vi "arrays.vi"() -> ()   [LabVIEW 2023]
panel:
  out "Waveform Chart":cluster{dbl, dbl}(graph)
  in  "stop":bool
  out "Waveform Graph":dbl[](graph)
  out "Array 4":dbl[][](array[numeric])
  out "Array 3":dbl[](array[numeric])
  in  "Array 2":dbl[](array[numeric])
  out "Array":dbl[](array[numeric])
  out "x+y 4":dbl[](array[numeric])
  out "x+y 3":dbl[](array[numeric])
  out "x+y 2":dbl[](array[numeric])
  out "x+y":dbl
  out "initialized array":dbl[][](array[numeric])
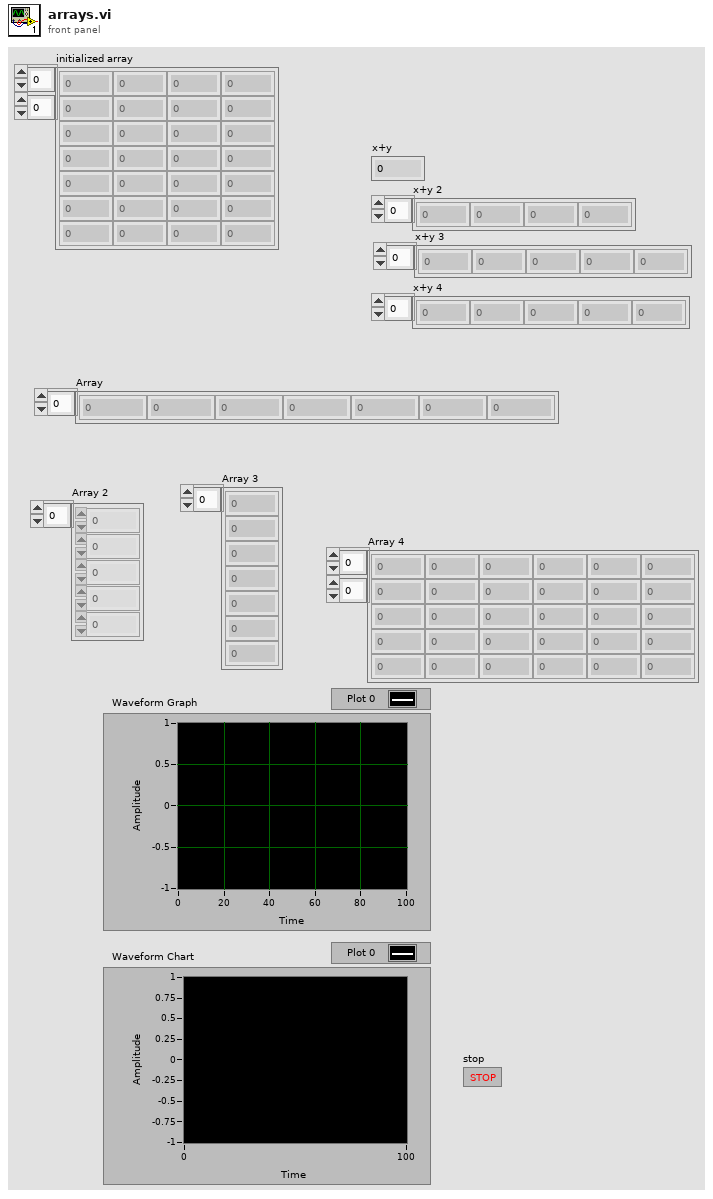
[diagram p1: front panel]
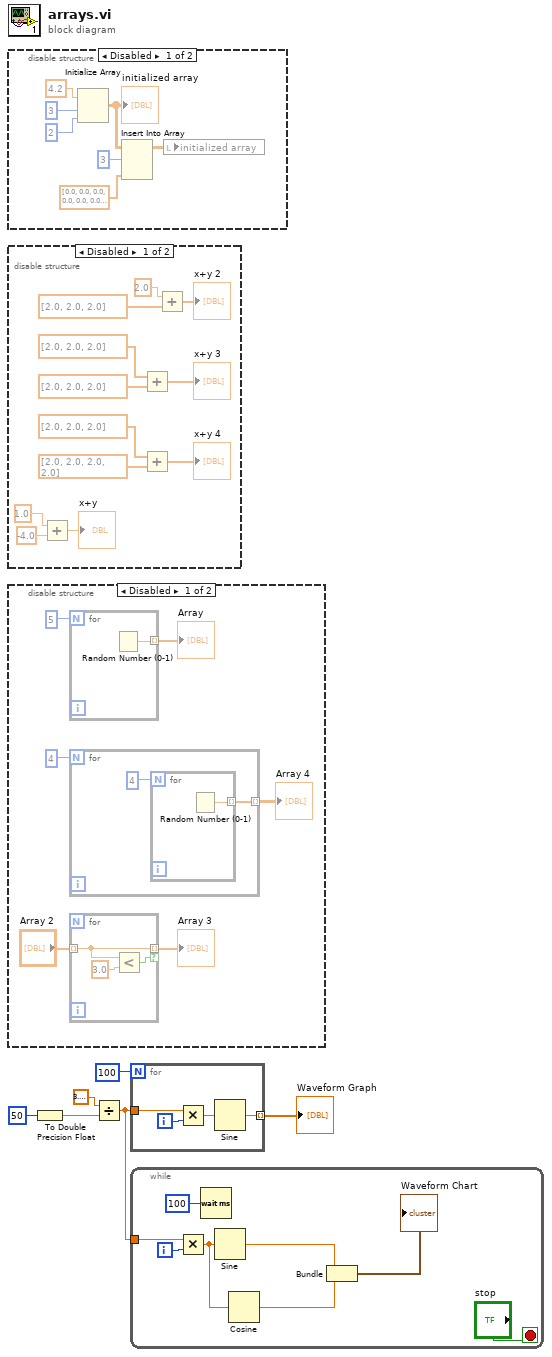
[diagram p0: block diagram]
diagram:
  n1 = disable-structure shown="Disabled" {
    frame Disabled {
      n2 = Initialize Array(4.2 ("element"), 3 ("dimension size"), 2 ("dimension size")) -> (w10:dbl[][])
      "initialized array" <- w10
      n3 = Insert Into Array(array=w10, index (row)=3, new element=dbl[] [0.0, 0.0, 0.0, 0.0, 0.0, 0.0, 0.0, 0.0, 0.0, 0.0, 0.0, 0.0, 0.0, 0.0, 0.0, 0.0, 0.0, 0.0, 0.0, 0.0, 0.0, 0.0, 0.0, 0.0, 0.0, 0.0, 0.0, 0.0, 0.0, 0.0, 0.0, 0.0, 0.0, 0.0, 34.0] ("new element/subarray")) -> (w7:dbl[][])  [unwired: 1 in]
      n4 = local write "initialized array"(w7) -> ()
    }
    frame Enabled {
    }
  }
  n5 = disable-structure shown="Disabled" {
    frame Disabled {
      n6 = Add(x=1.0, y=-4.0) -> (x+y=→"x+y":dbl)
      n7 = Add(x=dbl[] [2.0, 2.0, 2.0], y=dbl[] [2.0, 2.0, 2.0]) -> (x+y=→"x+y 3":dbl[])
      n8 = Add(x=dbl[] [2.0, 2.0, 2.0], y=dbl[] [2.0, 2.0, 2.0, 2.0]) -> (x+y=→"x+y 4":dbl[])
      n9 = Add(x=2.0, y=dbl[] [2.0, 2.0, 2.0]) -> (x+y=→"x+y 2":dbl[])
    }
    frame Enabled {
    }
  }
  n10 = disable-structure shown="Disabled" {
    frame Disabled {
      n11 = for {
        N: 5 -> [_]
        tunnel: [w38] -> w30 mode=indexing
        n12 = Random Number (0-1)() -> (number: 0 to 1=w38:dbl)
      }
      "Array" <- w30
      n13 = for {
        N: 4 -> [_]
        tunnel: [w32] -> w26 mode=indexing
        n14 = for {
          N: 4 -> [_]
          tunnel: [w34] -> w32 mode=indexing
          n15 = Random Number (0-1)() -> (number: 0 to 1=w34:dbl)
        }
      }
      "Array 4" <- w26
      n16 = for {
        tunnel: "Array 2" -> [w36] mode=indexing
        tunnel: [w36] -> w28 mode=indexing if=w35
        n17 = Less?(x=w36, y=3.0) -> (x < y?=w35:bool)
      }
      "Array 3" <- w28
    }
    frame Enabled {
    }
  }
  n18 = To Double Precision Float(number=50) -> (double precision float=w4:dbl)
  n19 = Divide(x=3.141592653589793, y=w4) -> (x/y=w1:dbl)
  n20 = for {
    N: 100 -> [_]
    tunnel: w1 -> [w41]
    tunnel: [w39] -> w2 mode=indexing
    i -> [w42]
    n21 = Multiply(x=w41, y=w42) -> (x*y=w40:dbl)
    n22 = Sine(x=w40) -> (sin(x)=w39:dbl)
  }
  "Waveform Graph" <- w2
  n23 = while {
    tunnel: w1 -> [w48]
    i -> [w49]
    stop <- "stop" stop-if-true
    n24 = Multiply(x=w48, y=w49) -> (x*y=w46:dbl)
    n25 = Wait (ms)(milliseconds to wait=u32 100) -> ()  [unwired: 1 out]
    n26 = Sine(x=w46) -> (sin(x)=w45:dbl)
    n27 = Cosine(x=w46) -> (cos(x)=w44:dbl)
    n28 = Bundle(w45, w44) -> (→"Waveform Chart":cluster{dbl, dbl})  [unwired: 1 in]
  }
